vi "Mem_DataToU8Array.vi"(8 "error in (no error)":errorcluster, 10 "Payload":variant, 11 "AddrQueueIn":refnum<queue>) -> (0 "error out":errorcluster, 1 "Supported Type?":bool, 2 "ByteArray":u8[](array[numeric]), 3 "AddrQueueOut":refnum<queue>)   [LabVIEW 2019, in "Memory Data Access.lvlib"]
uses:
  Memory Data Access.lvlib
  <vilib>/Utility/Data Type/Type Definitions/Data Type.ctl
  Global/Global.vi
  <vilib>/Utility/Data Type/NI_Data Type.lvlib
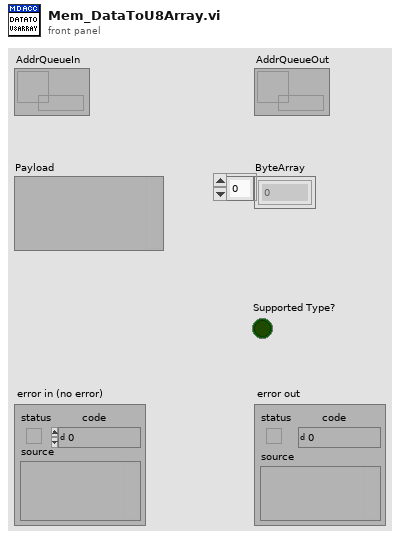
[diagram p1: front panel]
types:
  T1 = typedef "NI_Data Type.lvlib/Data Type.ctl" = enum8{"Invalid Type", "Void", "I8", "I16", "I32", "I64", "U8", "U16", "U32", "U64", "Single Float", "Double Float", "Extended Float", "Single Complex", "Double Complex", "Extended Complex", "Enum U8", "Enum U16", "Enum U32", "Enum U64", "Single Float With Unit", "Double Float With Unit", "Extended Float With Unit", "Single Complex with Unit", "Double Complex with Unit", "Extended Complex with Unit", "Boolean", "String", "Path", "Picture", "Tag", "Array", "Cluster", "Variant", "LV Variant", "Waveform", "Timestamp", "Digital Waveform", "Digital Data", "ExpressData", "Refnum", "External Data", "VI", "Poly VI", "LabVIEW Class Instance", "Fixed Point", "Set Collection", "Map Collection"}
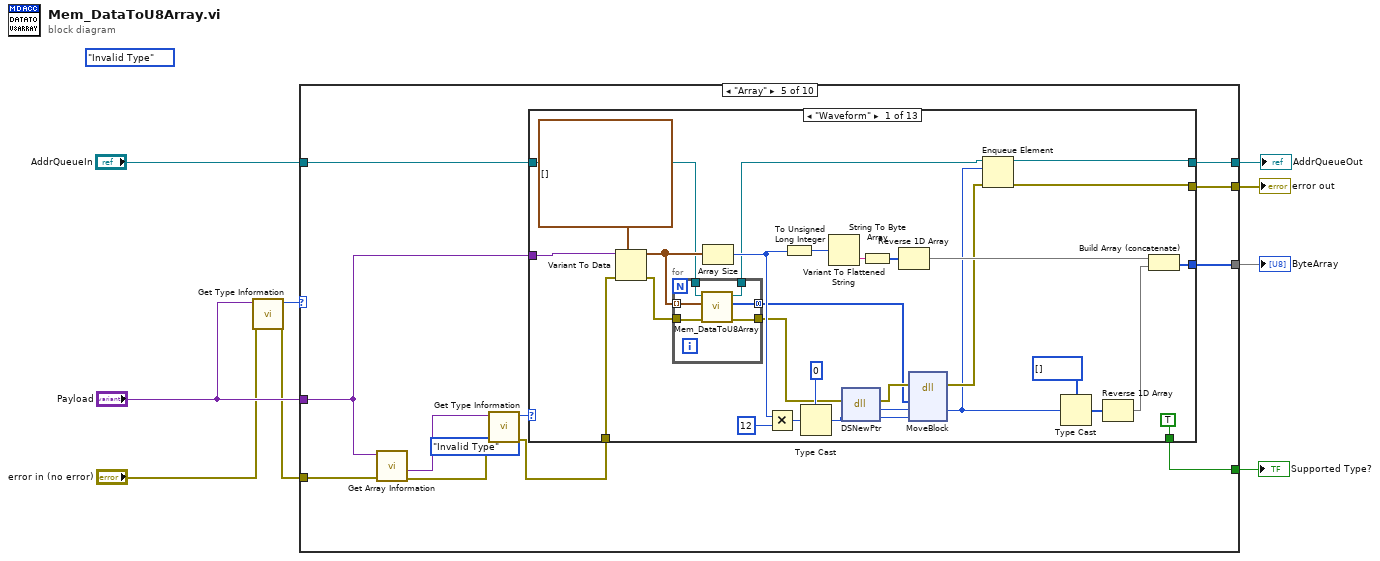
[diagram p0: block diagram]
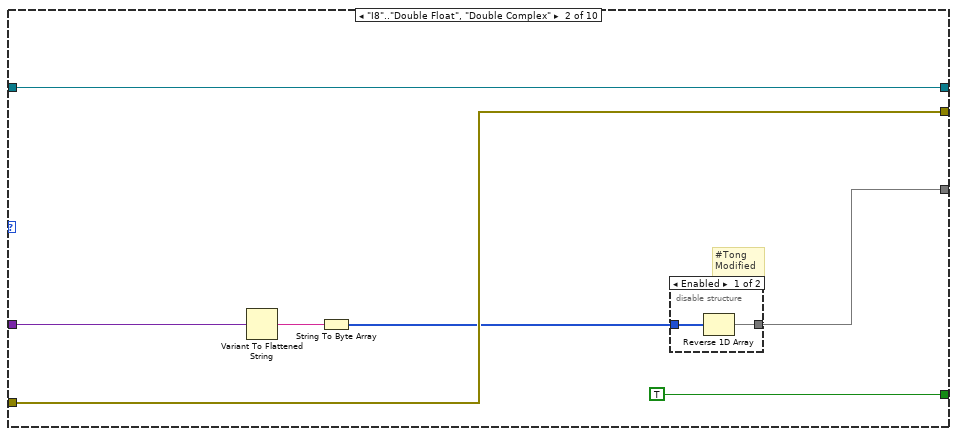
[diagram p3: hidden frame]
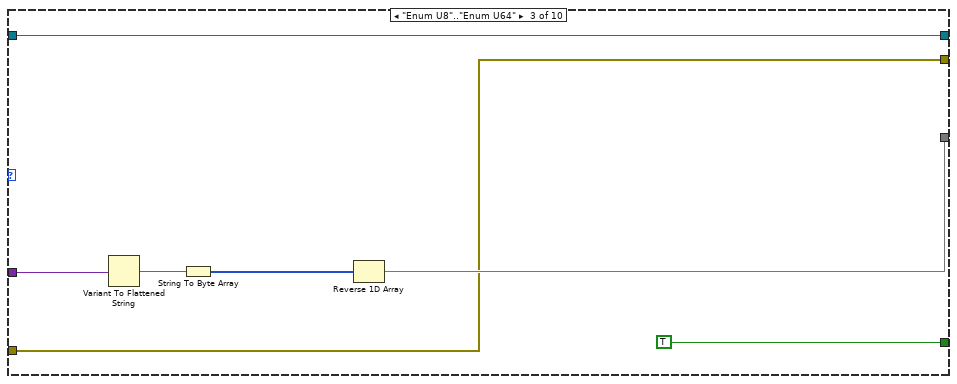
[diagram p5: hidden frame]
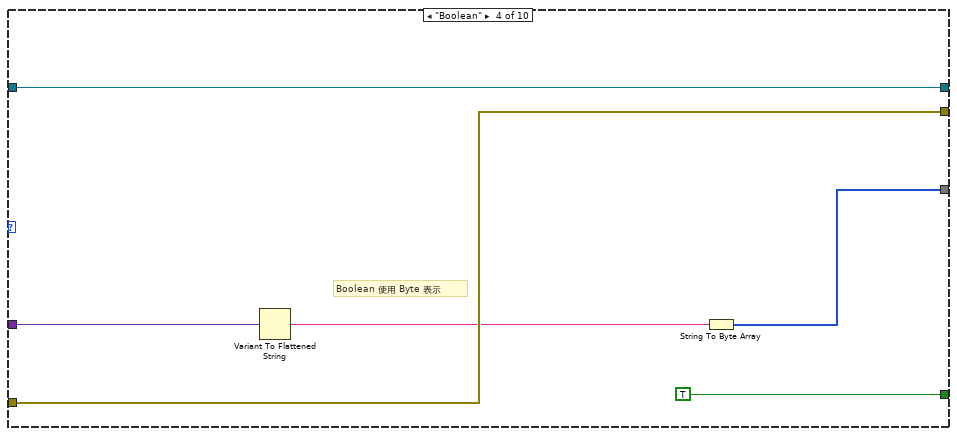
[diagram p6: hidden frame]
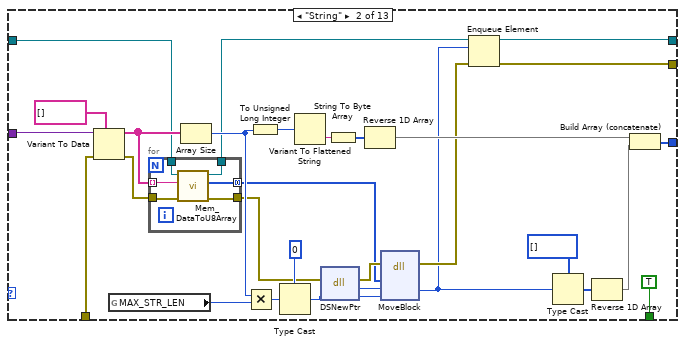
[diagram p7: hidden frame]
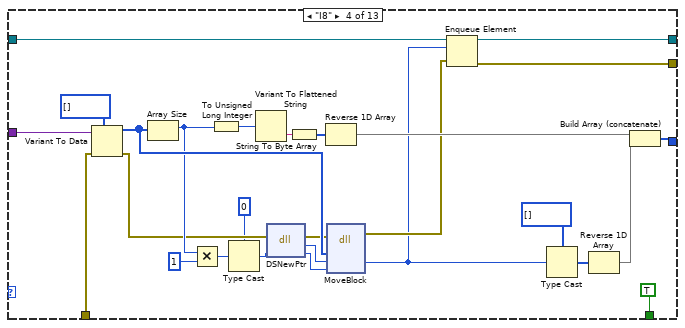
[diagram p9: hidden frame]
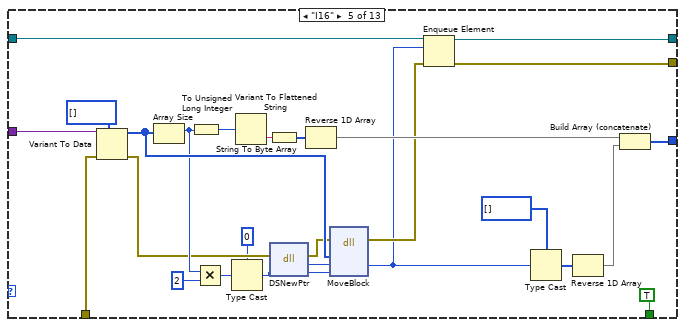
[diagram p10: hidden frame]
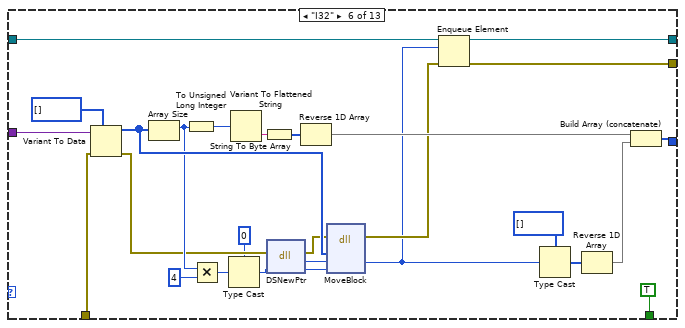
[diagram p11: hidden frame]
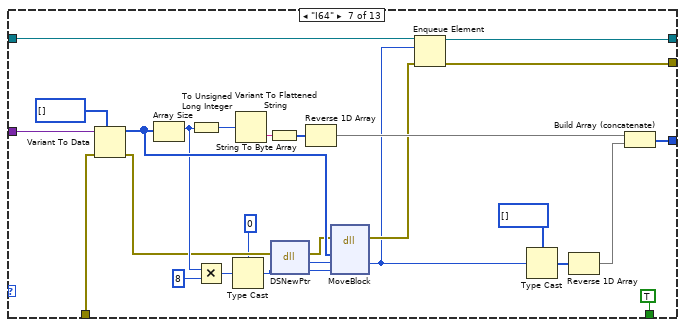
[diagram p12: hidden frame]
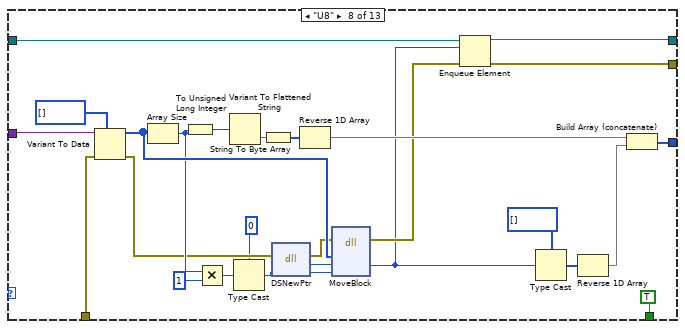
[diagram p13: hidden frame]
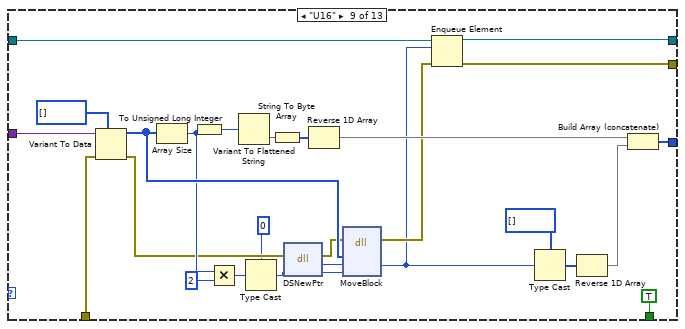
[diagram p14: hidden frame]
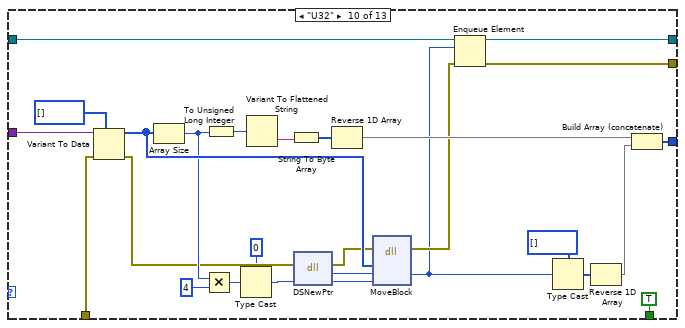
[diagram p15: hidden frame]
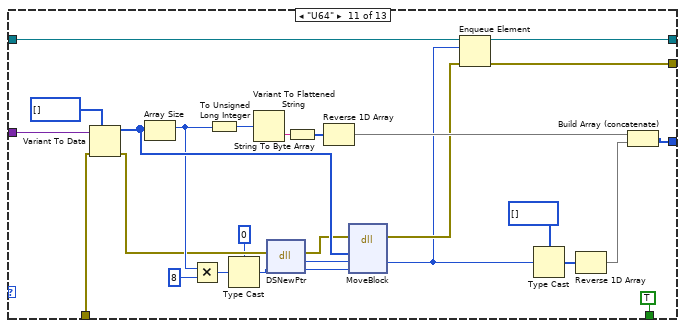
[diagram p16: hidden frame]
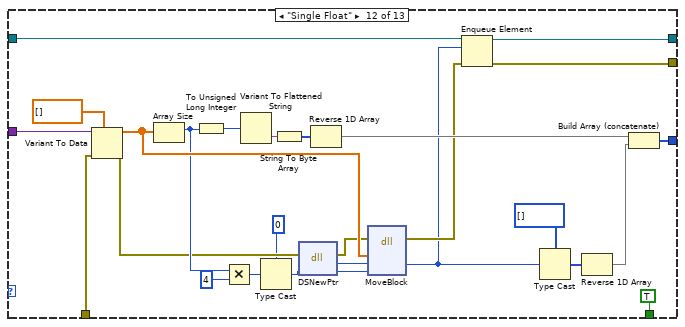
[diagram p17: hidden frame]
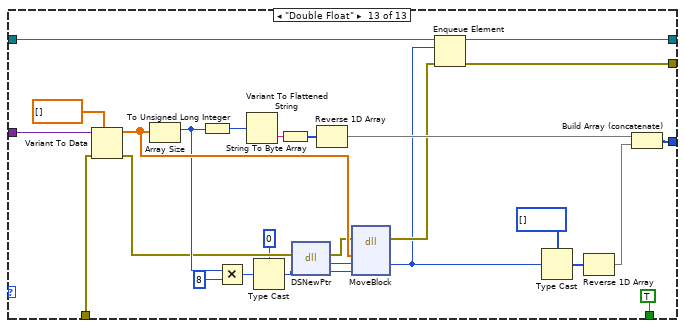
[diagram p18: hidden frame]
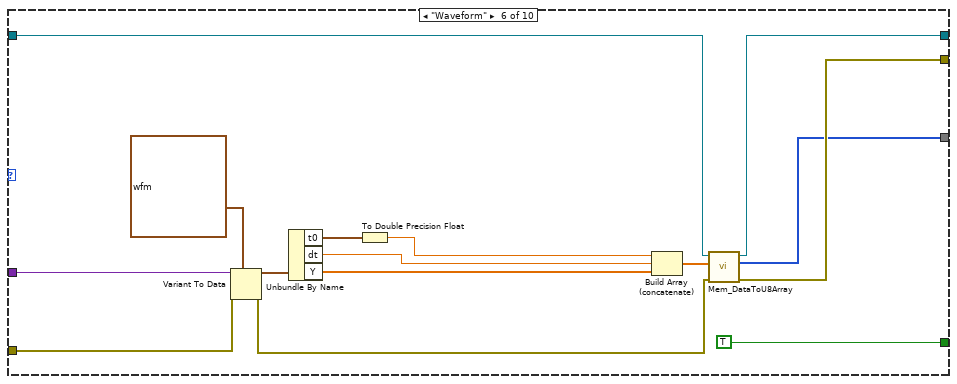
[diagram p19: hidden frame]
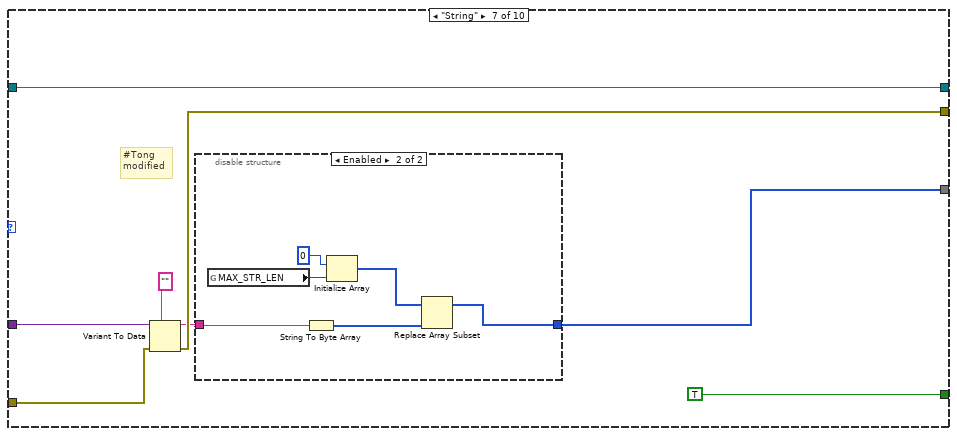
[diagram p20: hidden frame]
diagram:
  (unwired) Data_Type."Invalid Type" ("Type")
  n1 = call <vilib>:"Get Type Information.vi"("error in (no error)"="error in (no error)", "variant"="Payload") -> ("error out"=w3:errorcluster, "type"=w5:T1)  [unwired: 5 in, 3 out]
  n2 = case shown="\"Array\"" w5 {
    tunnel: w3 -> [w11 w18 w24 w34 w42 w396 w407 w427 w436 w448]
    tunnel: [w11 w18 w24 w34 w44 w393 w408 w428 w437 w449] -> w9
    tunnel: [_ w13 w25 w30 w45 w392 w410 w423 w439 w453] -> w8
    tunnel: "Payload" -> [_ w16 w27 w32 w43 w403 w411 w431 w440 w456]
    tunnel: [_ TRUE TRUE ("Supported Type?") TRUE w35 TRUE TRUE TRUE TRUE w451] -> w7
    tunnel: "AddrQueueIn" -> [w10 w12 w22 w29 w38 w391 w405 w422 w433 w447]
    tunnel: [w10 w12 w22 w29 w37 w390 w405 w422 w433 w446] -> w1
    frame "Invalid Type", Default {
    }
    frame "I8".."Double Float", "Double Complex" {
      # "#Tong\nModified"
      n3 = Variant To Flattened String(Variant=w16) -> (data string=w15:string)  [unwired: 1 out]
      n4 = String To Byte Array(string=w15) -> (unsigned byte array=w14:u8[])
      n5 = disable-structure shown="Enabled" {
        disable-tunnel: w14 -> [w20 w21]
        disable-tunnel: [w19 w21] -> w13
        frame Enabled {
          n6 = Reverse 1D Array(array=w20) -> (reversed array=w19:u8[])
        }
        frame Disabled {
        }
      }
    }
    frame "Enum U8".."Enum U64" {
      n7 = Variant To Flattened String(Variant=w27) -> (data string=w28:string)  [unwired: 1 out]
      n8 = String To Byte Array(string=w28) -> (unsigned byte array=w26:u8[])
      n9 = Reverse 1D Array(array=w26) -> (reversed array=w25:u8[])
    }
    frame "Boolean" {
      # "Boolean 使用 Byte 表示"
      n10 = Variant To Flattened String(Variant=w32) -> (data string=w31:string)  [unwired: 1 out]
      n11 = String To Byte Array(string=w31) -> (unsigned byte array=w30:u8[])
    }
    frame "Array" {
      (unwired) Data_Type."Invalid Type" ("type")
      n12 = call <vilib>:"Get Array Information.vi"("error in (no error)"=w42, "variant"=w43) -> ("error out"=w36:errorcluster, "array element data type"=w40:variant)  [unwired: 6 in, 2 out]
      n13 = call <vilib>:"Get Type Information.vi"("error in (no error)"=w36, "variant"=w40) -> ("error out"=w39:errorcluster, "type"=w41:T1)  [unwired: 5 in, 3 out]
      n14 = case shown="\"Waveform\"" w41 {
        tunnel: [w56 w95 _ w126 w154 w181 w208 w234 w261 w288 w315 w342 w369] -> w45
        tunnel: w43 -> [w55 w96 _ w128 w155 w182 w209 w236 w263 w291 w317 w344 w371]
        tunnel: w39 -> [w54 w94 w118 w127 w153 w180 w207 w235 w262 w290 w316 w343 w370]
        tunnel: [w49 w86 w118 w122 w150 w176 w202 w229 w257 w285 w311 w338 w366] -> w44
        tunnel: w38 -> [w48 w85 w119 w125 w152 w179 w206 w233 w260 w287 w314 w341 w368]
        tunnel: [w53 w88 w119 w124 w151 w178 w205 w232 w259 w283 w313 w340 w365] -> w37
        tunnel: [TRUE ("Supported Type?") TRUE ("Supported Type?") _ TRUE ("Supported Type?") TRUE ("Supported Type?") TRUE ("Supported Type?") TRUE ("Supported Type?") TRUE ("Supported Type?") TRUE ("Supported Type?") TRUE ("Supported Type?") TRUE ("Supported Type?") TRUE ("Supported Type?") TRUE ("Supported Type?")] -> w35
        frame "Waveform" {
          n15 = Variant To Data(error in=w54, type=waveform(dbl)[] [], Variant=w55) -> (data=w60:waveform(dbl)[], error out=w59:errorcluster)
          n16 = for {
            tunnel: w60 -> [w81] mode=indexing
            tunnel: w59 -> [w80]
            tunnel: [w79] -> w57 mode=concatenating
            tunnel: [w78] -> w58
            tunnel: w48 -> [w77]
            tunnel: [w76] -> w47
            n17 = call "Mem_DataToU8Array.vi"("error in (no error)"=w80, "Payload"=w81, "AddrQueueIn"=w77) -> ("error out"=w78:errorcluster, "ByteArray"=w79:u8[], "AddrQueueOut"=w76:refnum<queue>)  [unwired: 5 in, 1 out]
          }
          n18 = Array Size(array=w60) -> (size(s)=w71:i32)
          n19 = Multiply(x=w71, y=12) -> (x*y=w72:i32)
          n20 = To Unsigned Long Integer(number=w71) -> (unsigned 32bit integer=w68:u32)
          n21 = Type Cast(type=u32 0, x=w72) -> (*(type *) &x=w73:u32)
          n22 = Variant To Flattened String(Variant=w68) -> (data string=w67:string)  [unwired: 1 out]
          n23 = dll-call lib="LabVIEW" fn="DSNewPtr"(error in=w58, "size"=w73) -> (error out=w64:errorcluster, "return type"=w74:u64, "size"=w75:u32)  [unwired: 2 in, 1 out]
          n24 = String To Byte Array(string=w67) -> (unsigned byte array=w69:u8[])
          n25 = Reverse 1D Array(array=w69) -> (reversed array=w70:u8[])
          n26 = dll-call lib="LabVIEW" fn="MoveBlock"(error in=w64, "PointerSRC"=w57, "PointerDEST"=w74, "size"=w75) -> (error out=w51:errorcluster, "PointerDEST"=w50:u64)  [unwired: 5 in, 1 out]
          n27 = Enqueue Element(queue=w47, element=w50, error in (no error)=w51) -> (queue out=w53:refnum<queue>, error out=w49:errorcluster)  [unwired: 1 in, 1 out]
          n28 = Type Cast(type=u8[] [], x=w50) -> (*(type *) &x=w66:u8[])
          n29 = Reverse 1D Array(array=w66) -> (reversed array=w65:u8[])
          n30 = Build Array (concatenate)(w70, w65) -> (w56:u8[])
        }
        frame "String" {
          n31 = Variant To Data(error in=w94, type=string[] [], Variant=w96) -> (data=w93:string[], error out=w92:errorcluster)
          n32 = global read "Global.vi" "MAX_STR_LEN"() -> (w89:i32)
          n33 = for {
            tunnel: w93 -> [w117] mode=indexing
            tunnel: w92 -> [w116]
            tunnel: [w115] -> w90 mode=concatenating
            tunnel: [w114] -> w91
            tunnel: w85 -> [w113]
            tunnel: [w112] -> w83
            n34 = call "Mem_DataToU8Array.vi"("error in (no error)"=w116, "Payload"=w117, "AddrQueueIn"=w113) -> ("error out"=w114:errorcluster, "ByteArray"=w115:u8[], "AddrQueueOut"=w112:refnum<queue>)  [unwired: 5 in, 1 out]
          }
          n35 = Array Size(array=w93) -> (size(s)=w107:i32)
          n36 = Multiply(x=w107, y=w89) -> (x*y=w108:i32)
          n37 = To Unsigned Long Integer(number=w107) -> (unsigned 32bit integer=w104:u32)
          n38 = Type Cast(type=u32 0, x=w108) -> (*(type *) &x=w109:u32)
          n39 = Variant To Flattened String(Variant=w104) -> (data string=w103:string)  [unwired: 1 out]
          n40 = dll-call lib="LabVIEW" fn="DSNewPtr"(error in=w91, "size"=w109) -> (error out=w100:errorcluster, "return type"=w110:u64, "size"=w111:u32)  [unwired: 2 in, 1 out]
          n41 = String To Byte Array(string=w103) -> (unsigned byte array=w105:u8[])
          n42 = Reverse 1D Array(array=w105) -> (reversed array=w106:u8[])
          n43 = dll-call lib="LabVIEW" fn="MoveBlock"(error in=w100, "PointerSRC"=w90, "PointerDEST"=w110, "size"=w111) -> (error out=w87:errorcluster, "PointerDEST"=w84:u64)  [unwired: 5 in, 1 out]
          n44 = Enqueue Element(queue=w83, element=w84, error in (no error)=w87) -> (queue out=w88:refnum<queue>, error out=w86:errorcluster)  [unwired: 1 in, 1 out]
          n45 = Type Cast(type=u8[] [], x=w84) -> (*(type *) &x=w102:u8[])
          n46 = Reverse 1D Array(array=w102) -> (reversed array=w101:u8[])
          n47 = Build Array (concatenate)(w106, w101) -> (w95:u8[])
        }
        frame "Invalid Type", Default {
        }
        frame "I8" {
          n48 = Variant To Data(error in=w127, type=i8[] [], Variant=w128) -> (data=w144:i8[], error out=w136:errorcluster)
          n49 = Array Size(array=w144) -> (size(s)=w141:i32)
          n50 = Multiply(x=w141, y=1) -> (x*y=w142:i32)
          n51 = To Unsigned Long Integer(number=w141) -> (unsigned 32bit integer=w138:u32)
          n52 = Type Cast(type=u32 0, x=w142) -> (*(type *) &x=w143:u32)
          n53 = Variant To Flattened String(Variant=w138) -> (data string=w137:string)  [unwired: 1 out]
          n54 = dll-call lib="LabVIEW" fn="DSNewPtr"(error in=w136, "size"=w143) -> (error out=w133:errorcluster, "return type"=w145:u64, "size"=w146:u32)  [unwired: 2 in, 1 out]
          n55 = String To Byte Array(string=w137) -> (unsigned byte array=w139:u8[])
          n56 = Reverse 1D Array(array=w139) -> (reversed array=w140:u8[])
          n57 = dll-call lib="LabVIEW" fn="MoveBlock"(error in=w133, "PointerSRC"=w144, "PointerDEST"=w145, "size"=w146) -> (error out=w123:errorcluster, "PointerDEST"=w121:u64)  [unwired: 5 in, 1 out]
          n58 = Enqueue Element(queue=w125, element=w121, error in (no error)=w123) -> (queue out=w124:refnum<queue>, error out=w122:errorcluster)  [unwired: 1 in, 1 out]
          n59 = Type Cast(type=u8[] [], x=w121) -> (*(type *) &x=w135:u8[])
          n60 = Reverse 1D Array(array=w135) -> (reversed array=w134:u8[])
          n61 = Build Array (concatenate)(w140, w134) -> (w126:u8[])
        }
        frame "I16" {
          n62 = Variant To Data(error in=w153, type=i16[] [], Variant=w155) -> (data=w171:i16[], error out=w163:errorcluster)
          n63 = Array Size(array=w171) -> (size(s)=w168:i32)
          n64 = To Unsigned Long Integer(number=w168) -> (unsigned 32bit integer=w165:u32)
          n65 = Multiply(x=w168, y=2) -> (x*y=w169:i32)
          n66 = Type Cast(type=u32 0, x=w169) -> (*(type *) &x=w170:u32)
          n67 = Variant To Flattened String(Variant=w165) -> (data string=w164:string)  [unwired: 1 out]
          n68 = String To Byte Array(string=w164) -> (unsigned byte array=w166:u8[])
          n69 = dll-call lib="LabVIEW" fn="DSNewPtr"(error in=w163, "size"=w170) -> (error out=w160:errorcluster, "return type"=w172:u64, "size"=w173:u32)  [unwired: 2 in, 1 out]
          n70 = Reverse 1D Array(array=w166) -> (reversed array=w167:u8[])
          n71 = dll-call lib="LabVIEW" fn="MoveBlock"(error in=w160, "PointerSRC"=w171, "PointerDEST"=w172, "size"=w173) -> (error out=w149:errorcluster, "PointerDEST"=w148:u64)  [unwired: 5 in, 1 out]
          n72 = Enqueue Element(queue=w152, element=w148, error in (no error)=w149) -> (queue out=w151:refnum<queue>, error out=w150:errorcluster)  [unwired: 1 in, 1 out]
          n73 = Type Cast(type=u8[] [], x=w148) -> (*(type *) &x=w162:u8[])
          n74 = Reverse 1D Array(array=w162) -> (reversed array=w161:u8[])
          n75 = Build Array (concatenate)(w167, w161) -> (w154:u8[])
        }
        frame "I32" {
          n76 = Variant To Data(error in=w180, type=i32[] [], Variant=w182) -> (data=w198:i32[], error out=w190:errorcluster)
          n77 = Array Size(array=w198) -> (size(s)=w195:i32)
          n78 = To Unsigned Long Integer(number=w195) -> (unsigned 32bit integer=w192:u32)
          n79 = Multiply(x=w195, y=4) -> (x*y=w196:i32)
          n80 = Type Cast(type=u32 0, x=w196) -> (*(type *) &x=w197:u32)
          n81 = Variant To Flattened String(Variant=w192) -> (data string=w191:string)  [unwired: 1 out]
          n82 = String To Byte Array(string=w191) -> (unsigned byte array=w193:u8[])
          n83 = dll-call lib="LabVIEW" fn="DSNewPtr"(error in=w190, "size"=w197) -> (error out=w187:errorcluster, "return type"=w199:u64, "size"=w200:u32)  [unwired: 2 in, 1 out]
          n84 = Reverse 1D Array(array=w193) -> (reversed array=w194:u8[])
          n85 = dll-call lib="LabVIEW" fn="MoveBlock"(error in=w187, "PointerSRC"=w198, "PointerDEST"=w199, "size"=w200) -> (error out=w177:errorcluster, "PointerDEST"=w175:u64)  [unwired: 5 in, 1 out]
          n86 = Enqueue Element(queue=w179, element=w175, error in (no error)=w177) -> (queue out=w178:refnum<queue>, error out=w176:errorcluster)  [unwired: 1 in, 1 out]
          n87 = Type Cast(type=u8[] [], x=w175) -> (*(type *) &x=w189:u8[])
          n88 = Reverse 1D Array(array=w189) -> (reversed array=w188:u8[])
          n89 = Build Array (concatenate)(w194, w188) -> (w181:u8[])
        }
        frame "I64" {
          n90 = Variant To Data(error in=w207, type=i64[] [], Variant=w209) -> (data=w225:i64[], error out=w217:errorcluster)
          n91 = Array Size(array=w225) -> (size(s)=w222:i32)
          n92 = To Unsigned Long Integer(number=w222) -> (unsigned 32bit integer=w219:u32)
          n93 = Multiply(x=w222, y=8) -> (x*y=w223:i32)
          n94 = Type Cast(type=u32 0, x=w223) -> (*(type *) &x=w224:u32)
          n95 = Variant To Flattened String(Variant=w219) -> (data string=w218:string)  [unwired: 1 out]
          n96 = String To Byte Array(string=w218) -> (unsigned byte array=w220:u8[])
          n97 = dll-call lib="LabVIEW" fn="DSNewPtr"(error in=w217, "size"=w224) -> (error out=w214:errorcluster, "return type"=w226:u64, "size"=w227:u32)  [unwired: 2 in, 1 out]
          n98 = Reverse 1D Array(array=w220) -> (reversed array=w221:u8[])
          n99 = dll-call lib="LabVIEW" fn="MoveBlock"(error in=w214, "PointerSRC"=w225, "PointerDEST"=w226, "size"=w227) -> (error out=w204:errorcluster, "PointerDEST"=w203:u64)  [unwired: 5 in, 1 out]
          n100 = Enqueue Element(queue=w206, element=w203, error in (no error)=w204) -> (queue out=w205:refnum<queue>, error out=w202:errorcluster)  [unwired: 1 in, 1 out]
          n101 = Type Cast(type=u8[] [], x=w203) -> (*(type *) &x=w216:u8[])
          n102 = Reverse 1D Array(array=w216) -> (reversed array=w215:u8[])
          n103 = Build Array (concatenate)(w221, w215) -> (w208:u8[])
        }
        frame "U8" {
          n104 = Variant To Data(error in=w235, type=u8[] [], Variant=w236) -> (data=w252:u8[], error out=w244:errorcluster)
          n105 = Array Size(array=w252) -> (size(s)=w249:i32)
          n106 = To Unsigned Long Integer(number=w249) -> (unsigned 32bit integer=w246:u32)
          n107 = Multiply(x=w249, y=1) -> (x*y=w250:i32)
          n108 = Variant To Flattened String(Variant=w246) -> (data string=w245:string)  [unwired: 1 out]
          n109 = Type Cast(type=u32 0, x=w250) -> (*(type *) &x=w251:u32)
          n110 = String To Byte Array(string=w245) -> (unsigned byte array=w247:u8[])
          n111 = dll-call lib="LabVIEW" fn="DSNewPtr"(error in=w244, "size"=w251) -> (error out=w241:errorcluster, "return type"=w253:u64, "size"=w254:u32)  [unwired: 2 in, 1 out]
          n112 = Reverse 1D Array(array=w247) -> (reversed array=w248:u8[])
          n113 = dll-call lib="LabVIEW" fn="MoveBlock"(error in=w241, "PointerSRC"=w252, "PointerDEST"=w253, "size"=w254) -> (error out=w231:errorcluster, "PointerDEST"=w230:u64)  [unwired: 5 in, 1 out]
          n114 = Enqueue Element(queue=w233, element=w230, error in (no error)=w231) -> (queue out=w232:refnum<queue>, error out=w229:errorcluster)  [unwired: 1 in, 1 out]
          n115 = Type Cast(type=u8[] [], x=w230) -> (*(type *) &x=w243:u8[])
          n116 = Reverse 1D Array(array=w243) -> (reversed array=w242:u8[])
          n117 = Build Array (concatenate)(w248, w242) -> (w234:u8[])
        }
        frame "U16" {
          n118 = Variant To Data(error in=w262, type=u16[] [], Variant=w263) -> (data=w279:u16[], error out=w271:errorcluster)
          n119 = Array Size(array=w279) -> (size(s)=w276:i32)
          n120 = To Unsigned Long Integer(number=w276) -> (unsigned 32bit integer=w273:u32)
          n121 = Multiply(x=w276, y=2) -> (x*y=w277:i32)
          n122 = Variant To Flattened String(Variant=w273) -> (data string=w272:string)  [unwired: 1 out]
          n123 = Type Cast(type=u32 0, x=w277) -> (*(type *) &x=w278:u32)
          n124 = String To Byte Array(string=w272) -> (unsigned byte array=w274:u8[])
          n125 = dll-call lib="LabVIEW" fn="DSNewPtr"(error in=w271, "size"=w278) -> (error out=w268:errorcluster, "return type"=w280:u64, "size"=w281:u32)  [unwired: 2 in, 1 out]
          n126 = Reverse 1D Array(array=w274) -> (reversed array=w275:u8[])
          n127 = dll-call lib="LabVIEW" fn="MoveBlock"(error in=w268, "PointerSRC"=w279, "PointerDEST"=w280, "size"=w281) -> (error out=w258:errorcluster, "PointerDEST"=w256:u64)  [unwired: 5 in, 1 out]
          n128 = Enqueue Element(queue=w260, element=w256, error in (no error)=w258) -> (queue out=w259:refnum<queue>, error out=w257:errorcluster)  [unwired: 1 in, 1 out]
          n129 = Type Cast(type=u8[] [], x=w256) -> (*(type *) &x=w270:u8[])
          n130 = Reverse 1D Array(array=w270) -> (reversed array=w269:u8[])
          n131 = Build Array (concatenate)(w275, w269) -> (w261:u8[])
        }
        frame "U32" {
          n132 = Variant To Data(error in=w290, type=u32[] [], Variant=w291) -> (data=w306:u32[], error out=w298:errorcluster)
          n133 = Array Size(array=w306) -> (size(s)=w303:i32)
          n134 = Multiply(x=w303, y=4) -> (x*y=w304:i32)
          n135 = To Unsigned Long Integer(number=w303) -> (unsigned 32bit integer=w300:u32)
          n136 = Type Cast(type=u32 0, x=w304) -> (*(type *) &x=w305:u32)
          n137 = Variant To Flattened String(Variant=w300) -> (data string=w299:string)  [unwired: 1 out]
          n138 = String To Byte Array(string=w299) -> (unsigned byte array=w301:u8[])
          n139 = dll-call lib="LabVIEW" fn="DSNewPtr"(error in=w298, "size"=w305) -> (error out=w295:errorcluster, "return type"=w307:u64, "size"=w308:u32)  [unwired: 2 in, 1 out]
          n140 = Reverse 1D Array(array=w301) -> (reversed array=w302:u8[])
          n141 = dll-call lib="LabVIEW" fn="MoveBlock"(error in=w295, "PointerSRC"=w306, "PointerDEST"=w307, "size"=w308) -> (error out=w286:errorcluster, "PointerDEST"=w284:u64)  [unwired: 5 in, 1 out]
          n142 = Enqueue Element(queue=w287, element=w284, error in (no error)=w286) -> (queue out=w283:refnum<queue>, error out=w285:errorcluster)  [unwired: 1 in, 1 out]
          n143 = Type Cast(type=u8[] [], x=w284) -> (*(type *) &x=w297:u8[])
          n144 = Reverse 1D Array(array=w297) -> (reversed array=w296:u8[])
          n145 = Build Array (concatenate)(w302, w296) -> (w288:u8[])
        }
        frame "U64" {
          n146 = Variant To Data(error in=w316, type=u64[] [], Variant=w317) -> (data=w333:u64[], error out=w325:errorcluster)
          n147 = Array Size(array=w333) -> (size(s)=w330:i32)
          n148 = Multiply(x=w330, y=8) -> (x*y=w331:i32)
          n149 = To Unsigned Long Integer(number=w330) -> (unsigned 32bit integer=w327:u32)
          n150 = Type Cast(type=u32 0, x=w331) -> (*(type *) &x=w332:u32)
          n151 = Variant To Flattened String(Variant=w327) -> (data string=w326:string)  [unwired: 1 out]
          n152 = dll-call lib="LabVIEW" fn="DSNewPtr"(error in=w325, "size"=w332) -> (error out=w322:errorcluster, "return type"=w334:u64, "size"=w335:u32)  [unwired: 2 in, 1 out]
          n153 = String To Byte Array(string=w326) -> (unsigned byte array=w328:u8[])
          n154 = Reverse 1D Array(array=w328) -> (reversed array=w329:u8[])
          n155 = dll-call lib="LabVIEW" fn="MoveBlock"(error in=w322, "PointerSRC"=w333, "PointerDEST"=w334, "size"=w335) -> (error out=w312:errorcluster, "PointerDEST"=w310:u64)  [unwired: 5 in, 1 out]
          n156 = Enqueue Element(queue=w314, element=w310, error in (no error)=w312) -> (queue out=w313:refnum<queue>, error out=w311:errorcluster)  [unwired: 1 in, 1 out]
          n157 = Type Cast(type=u8[] [], x=w310) -> (*(type *) &x=w324:u8[])
          n158 = Reverse 1D Array(array=w324) -> (reversed array=w323:u8[])
          n159 = Build Array (concatenate)(w329, w323) -> (w315:u8[])
        }
        frame "Single Float" {
          n160 = Variant To Data(error in=w343, type=sgl[] [], Variant=w344) -> (data=w360:sgl[], error out=w352:errorcluster)
          n161 = Array Size(array=w360) -> (size(s)=w357:i32)
          n162 = To Unsigned Long Integer(number=w357) -> (unsigned 32bit integer=w354:u32)
          n163 = Multiply(x=w357, y=4) -> (x*y=w358:i32)
          n164 = Variant To Flattened String(Variant=w354) -> (data string=w353:string)  [unwired: 1 out]
          n165 = Type Cast(type=u32 0, x=w358) -> (*(type *) &x=w359:u32)
          n166 = String To Byte Array(string=w353) -> (unsigned byte array=w355:u8[])
          n167 = dll-call lib="LabVIEW" fn="DSNewPtr"(error in=w352, "size"=w359) -> (error out=w349:errorcluster, "return type"=w361:u64, "size"=w362:u32)  [unwired: 2 in, 1 out]
          n168 = Reverse 1D Array(array=w355) -> (reversed array=w356:u8[])
          n169 = dll-call lib="LabVIEW" fn="MoveBlock"(error in=w349, "PointerSRC"=w360, "PointerDEST"=w361, "size"=w362) -> (error out=w339:errorcluster, "PointerDEST"=w337:u64)  [unwired: 5 in, 1 out]
          n170 = Enqueue Element(queue=w341, element=w337, error in (no error)=w339) -> (queue out=w340:refnum<queue>, error out=w338:errorcluster)  [unwired: 1 in, 1 out]
          n171 = Type Cast(type=u8[] [], x=w337) -> (*(type *) &x=w351:u8[])
          n172 = Reverse 1D Array(array=w351) -> (reversed array=w350:u8[])
          n173 = Build Array (concatenate)(w356, w350) -> (w342:u8[])
        }
        frame "Double Float" {
          n174 = Variant To Data(error in=w370, type=dbl[] [], Variant=w371) -> (data=w387:dbl[], error out=w379:errorcluster)
          n175 = Array Size(array=w387) -> (size(s)=w384:i32)
          n176 = To Unsigned Long Integer(number=w384) -> (unsigned 32bit integer=w381:u32)
          n177 = Multiply(x=w384, y=8) -> (x*y=w385:i32)
          n178 = Variant To Flattened String(Variant=w381) -> (data string=w380:string)  [unwired: 1 out]
          n179 = Type Cast(type=u32 0, x=w385) -> (*(type *) &x=w386:u32)
          n180 = String To Byte Array(string=w380) -> (unsigned byte array=w382:u8[])
          n181 = dll-call lib="LabVIEW" fn="DSNewPtr"(error in=w379, "size"=w386) -> (error out=w376:errorcluster, "return type"=w388:u64, "size"=w389:u32)  [unwired: 2 in, 1 out]
          n182 = Reverse 1D Array(array=w382) -> (reversed array=w383:u8[])
          n183 = dll-call lib="LabVIEW" fn="MoveBlock"(error in=w376, "PointerSRC"=w387, "PointerDEST"=w388, "size"=w389) -> (error out=w367:errorcluster, "PointerDEST"=w364:u64)  [unwired: 5 in, 1 out]
          n184 = Enqueue Element(queue=w368, element=w364, error in (no error)=w367) -> (queue out=w365:refnum<queue>, error out=w366:errorcluster)  [unwired: 1 in, 1 out]
          n185 = Type Cast(type=u8[] [], x=w364) -> (*(type *) &x=w378:u8[])
          n186 = Reverse 1D Array(array=w378) -> (reversed array=w377:u8[])
          n187 = Build Array (concatenate)(w383, w377) -> (w369:u8[])
        }
      }
    }
    frame "Waveform" {
      n188 = Variant To Data(error in=w396, type=waveform(dbl) {"t0"=timestamp(0 s since 1904-01-01), "dt"=1.0, "Y"=[]} ("Waveform"), Variant=w403) -> (data=w401:waveform(dbl), error out=w394:errorcluster)
      n189 = Unbundle By Name(w401) -> ("t0"=w399:timestamp, "dt"=w397:dbl, "Y"=w400:dbl[])
      n190 = To Double Precision Float(number=w399) -> (double precision float=w398:dbl)
      n191 = Build Array (concatenate)(w398, w397, w400) -> (w395:dbl[])
      n192 = call "Mem_DataToU8Array.vi"("error in (no error)"=w394, "Payload"=w395, "AddrQueueIn"=w391) -> ("error out"=w393:errorcluster, "ByteArray"=w392:u8[], "AddrQueueOut"=w390:refnum<queue>)  [unwired: 5 in, 1 out]
    }
    frame "String" {
      # "#Tong\nmodified"
      n193 = Variant To Data(error in=w407, type="" ("Waveform"), Variant=w411) -> (data=w406:string, error out=w408:errorcluster)
      n194 = disable-structure shown="Enabled" {
        disable-tunnel: [w415 w417] -> w410
        disable-tunnel: w406 -> [w414 w419]
        frame Disabled {
          n195 = String To Byte Array(string=w414) -> (unsigned byte array=w413:u8[])
          n196 = Variant To Flattened String(Variant=w413) -> (data string=w415:string)  [unwired: 1 out]
        }
        frame Enabled {
          n197 = global read "Global.vi" "MAX_STR_LEN"() -> (w416:i32)
          n198 = String To Byte Array(string=w419) -> (unsigned byte array=w418:u8[])
          n199 = Initialize Array(u8 0 ("*(type *) &x"), w416) -> (w420:u8[])
          n200 = Replace Array Subset(array=w420, new element=w418) -> (w417:u8[])  [unwired: 1 in]
        }
      }
    }
    frame "Timestamp" {
      n201 = Variant To Data(error in=w427, type=timestamp(0 s since 1904-01-01) ("Waveform"), Variant=w431) -> (data=w426:timestamp, error out=w428:errorcluster)
      n202 = To Double Precision Float(number=w426) -> (double precision float=w425:dbl)
      n203 = Variant To Flattened String(Variant=w425) -> (data string=w430:string)  [unwired: 1 out]
      n204 = String To Byte Array(string=w430) -> (unsigned byte array=w424:u8[])
      n205 = Reverse 1D Array(array=w424) -> (reversed array=w423:u8[])
    }
    frame "Path" {
      n206 = Variant To Data(error in=w436, type=path "" ("Waveform"), Variant=w440) -> (data=w435:path, error out=w437:errorcluster)
      n207 = Path To String(path=w435) -> (string=w434:string)
      n208 = disable-structure shown="Enabled" {
        disable-tunnel: [w443 w444] -> w439
        disable-tunnel: w434 -> [w442 w445]
        frame Disabled {
          n209 = Variant To Flattened String(Variant=w442) -> (data string=w443:string)  [unwired: 1 out]
        }
        frame Enabled {
          n210 = String To Byte Array(string=w445) -> (unsigned byte array=w444:u8[])
        }
      }
    }
    frame "Cluster" {
      n211 = call <userlib>:"Cluster to Array of VData__ogtk.vi"("error in (no error)"=w448, "Cluster"=w456) -> ("error out"=w450:errorcluster, "Array of VData"=w455:variant[])  [unwired: 8 in]
      n212 = for {
        tunnel: w455 -> [w463] mode=indexing
        tunnel: [w462] -> w454 mode=concatenating
        tunnel: [w461] -> w452 mode=indexing
        shift-right: [w459] -> w449
        shift-left: w450 -> [w460]
        tunnel: w447 -> [w458]
        tunnel: [w457] -> w446
        n213 = call "Mem_DataToU8Array.vi"("error in (no error)"=w460, "Payload"=w463, "AddrQueueIn"=w458) -> ("error out"=w459:errorcluster, "Supported Type?"=w461:bool, "ByteArray"=w462:u8[], "AddrQueueOut"=w457:refnum<queue>)  [unwired: 5 in]
      }
      n214 = Build Array (concatenate)(w454) -> (w453:u8[])
      n215 = And Array Elements(Boolean array=w452) -> (logical AND=w451:bool)
    }
  }
  "error out" <- w9
  "ByteArray" <- w8
  "Supported Type?" <- w7
  "AddrQueueOut" <- w1
